vi "Diff_Core.vi"(8 "error in (no error)":errorcluster, 9 "palette path 2":path, 11 "palette path  1":path) -> (0 "error out":errorcluster)   [LabVIEW 2017]
doc: "After you run the Create New Palette VI, run the Extract Palette Information VI to extract data from the palette file (.mnu). This VI displays the extracted data in the palette data cluster."
uses:
  <vilib>/Palette API/Palette Menu/Public Type Define/Palette type.ctl
  <vilib>/Palette API/Palette Menu/Palette Menu.lvlib
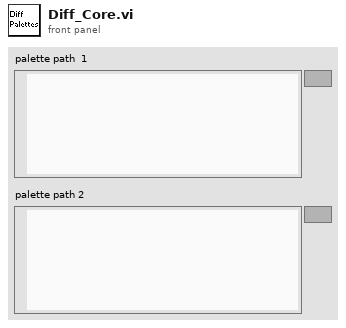
[diagram p1: front panel]
types:
  T1 = typedef "Palette Menu.lvlib/Palette type.ctl" = i32
  T2 = typedef "Palette Menu.lvlib/Palette Data.ctl" = cluster{"display name":string, "view format":T3, "palette width":i16, "items":T4, "256 color icon":picture, "B&W color icon":picture, "help information":T6, "palette description":string, "synchronize information":T7}
  T3 = typedef "Palette Menu.lvlib/View Format.ctl" = u16
  T4 = typedef "Palette Menu.lvlib/Items.ctl" = T5[]
  T5 = typedef "Palette Menu.lvlib/Item.ctl" = cluster{"item path":path, "library path (.lvlib)":path, "use default lvlib palette":bool, "short name":string, "place VI contents":bool, "hide synchronized item":bool, "reserve spot for synch item":bool, "configure when placing VI contents":bool}
  T6 = typedef "Palette Menu.lvlib/Help Info.ctl" = cluster{"help tag":string, "help file path ":path}
  T7 = typedef "Palette Menu.lvlib/Synchronize Info.ctl" = cluster{"synchronize with directory":bool, "synchronize directory path":path}
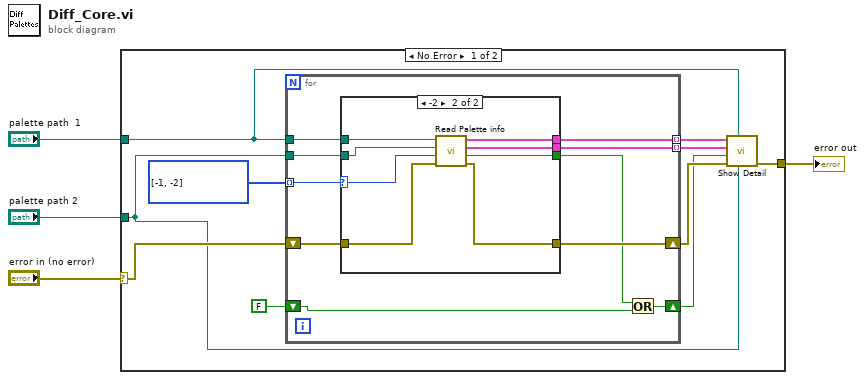
[diagram p0: block diagram]
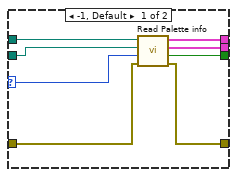
[diagram p2: hidden frame]
diagram:
  n1 = case shown="No Error" "error in (no error)" {
    selector: "error in (no error)" -> [w11 w41]
    tunnel: "palette path 2" -> [w5 _]
    tunnel: "palette path  1" -> [w6 _]
    tunnel: [w10 w41] -> w1
    frame No Error {
      w14 = T1[] [-1, -2] items=["Functions"=-1, "Controls"=-2] ("Array")
      n2 = for {
        tunnel: w6 -> [w24]
        tunnel: w5 -> [w23]
        tunnel: w14 -> [w22] mode=indexing
        shift-right: [w21] -> w12
        shift-left: w11 -> [w20]
        shift-right: [w19] -> w7
        shift-left: FALSE -> [w17]
        tunnel: [w16] -> w9 mode=indexing
        tunnel: [w15] -> w8 mode=indexing
        n3 = case shown="-2" w22 {
          selector: w22 -> [w29 w38]
          tunnel: w24 -> [w32 w40]
          tunnel: w20 -> [w31 w37]
          tunnel: w23 -> [w30 w39]
          tunnel: [w28 w36] -> w21
          tunnel: [w27 w33] -> w18
          tunnel: [w26 w35] -> w16
          tunnel: [w25 w34] -> w15
          frame -1, Default {
            n4 = call "Read Palette info.vi"("error in"=w31, "palette type"=w29, "palette path 2"=w30, "palette path  1"=w32) -> ("error out"=w28:errorcluster, "Palettes Different?"=w27:bool, "palette data 2"=w25:T2, "palette data 1"=w26:T2)  [unwired: 1 in, 3 out]
          }
          frame -2 {
            n5 = call "Read Palette info.vi"("error in"=w37, "palette type"=w38, "palette path 2"=w39, "palette path  1"=w40) -> ("error out"=w36:errorcluster, "Palettes Different?"=w33:bool, "palette data 2"=w34:T2, "palette data 1"=w35:T2)  [unwired: 1 in, 3 out]
          }
        }
        n6 = Or(x=w18, y=w17) -> (x .or. y?=w19:bool)
      }
      n7 = call "Show Detail.vi"("mnu file Path 2"=w5, "mnu file Path 1"=w6, "error in (no error)"=w12, "Palettes Different?"=w7, "Palette data array 2"=w8, "Palette data array 1"=w9) -> ("error out"=w10:errorcluster)  [unwired: 5 out]
    }
    frame Error {
    }
  }
  "error out" <- w1
